vi "Convert_Data.vi"(0 "I2C_Data":T3 {"Target_Specification"."Target_Address" format="%x"; "Target_Specification"."Target_Type" items=["10 Bit Address", "7 Bit Address"]; "Target_Specification"."Register_Address" format="%x"; "Read_Write" items=["ADD TARGET"]}, 5 "CSV_String_In":string, 11 "Error_In":errorcluster, 13 "Convert_Mode":T5=enum."Data_to_String") -> (4 "I2C_Data":T3 {"Target_Specification"."Target_Address" format="%x"; "Target_Specification"."Target_Type" items=["10 Bit Address", "7 Bit Address"]; "Target_Specification"."Register_Address" format="%x"; "Read_Write" items=["ADD TARGET"]}, 6 "CSV_String":string, 8 "Data":T1[](array[typedef]) {"Target_Type" items=["10 Bit Address", "7 Bit Address"]; "Selected_Register_Address" format="%x"; "Target_Address" format="%x"}, 15 "Error_Out":errorcluster)   [LabVIEW 2023]
uses:
  Controls/Convert_Mode.ctl
  Class/I2C/I2C.lvclass
  Controls/Control 5.ctl
  Controls/Menu_Ring.ctl
  Controls/Control 2.ctl
  Controls/Converted_Data.ctl
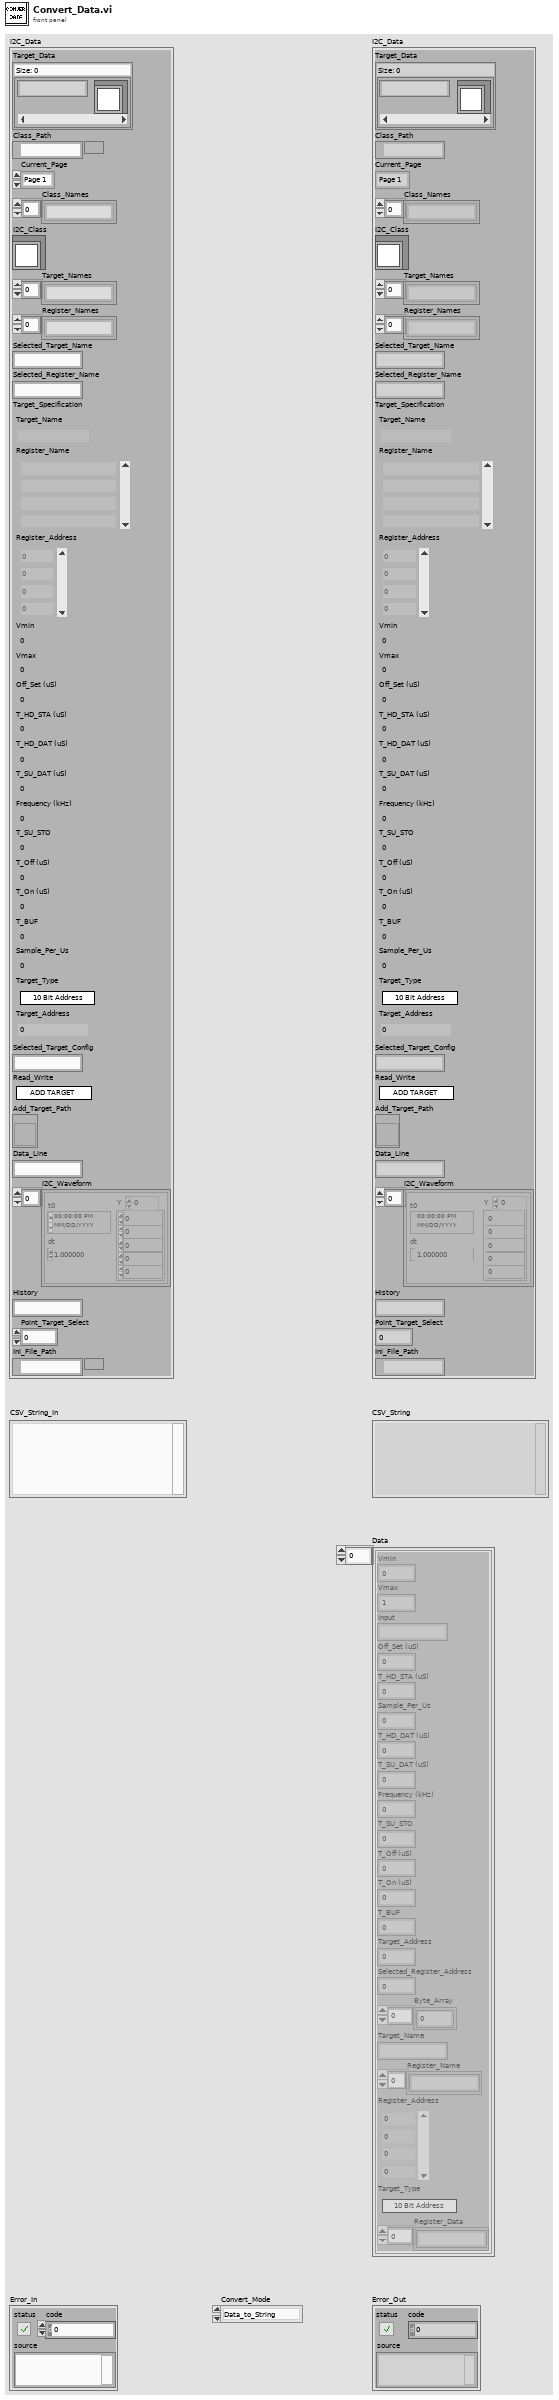
[diagram p1: front panel]
types:
  T1 = typedef "Converted_Data.ctl" = cluster{"Vmin":dbl, "Vmax":dbl, "Input":string, "Off_Set (uS)":dbl, "T_HD_STA (uS)":dbl, "Sample_Per_Us":dbl, "T_HD_DAT (uS)":dbl, "T_SU_DAT (uS)":dbl, "Frequency (kHz)":dbl, "T_SU_STO":dbl, "T_Off (uS)":dbl, "T_On (uS)":dbl, "T_BUF":dbl, "Target_Address":u16, "Selected_Register_Address":u8, "Byte_Array":u8[], "Target_Name":string, "Register_Name":string[], "Register_Address":u8[], "Target_Type":T2, "Register_Data":string[]}
  T2 = typedef "Menu_Ring.ctl" = u16
  T3 = typedef "Convert_Mode.ctl" = cluster{"Target_Data":map{string, refnum<class "I2C.lvclass">}, "Class_Path":path, "Current_Page":enum32{"Page 1", "Page 2"}, "Class_Names":string[], "I2C_Class":refnum<class "I2C.lvclass">, "Target_Names":string[], "Register_Names":string[], "Selected_Target_Name":string, "Selected_Register_Name":string, "Target_Specification":T4, "Selected_Target_Config":string, "Read_Write":T2, "Add_Target_Path":refnum<vi>, "Data_Line":string, "I2C_Waveform":waveform(dbl)[], "History":string, "Point_Target_Select":i32, "Ini_File_Path":path}
  T4 = typedef "Control 5.ctl" = cluster{"Target_Name":string, "Register_Name":string[], "Register_Address":u16[], "Vmin":dbl, "Vmax":dbl, "Off_Set (uS)":dbl, "T_HD_STA (uS)":dbl, "T_HD_DAT (uS)":dbl, "T_SU_DAT (uS)":dbl, "Frequency (kHz)":dbl, "T_SU_STO":dbl, "T_Off (uS)":dbl, "T_On (uS)":dbl, "T_BUF":dbl, "Sample_Per_Us":dbl, "Target_Type":T2, "Target_Address":u16}
  T5 = typedef "Control 2.ctl" = enum16{"String_To_Data", "Data_to_String"}
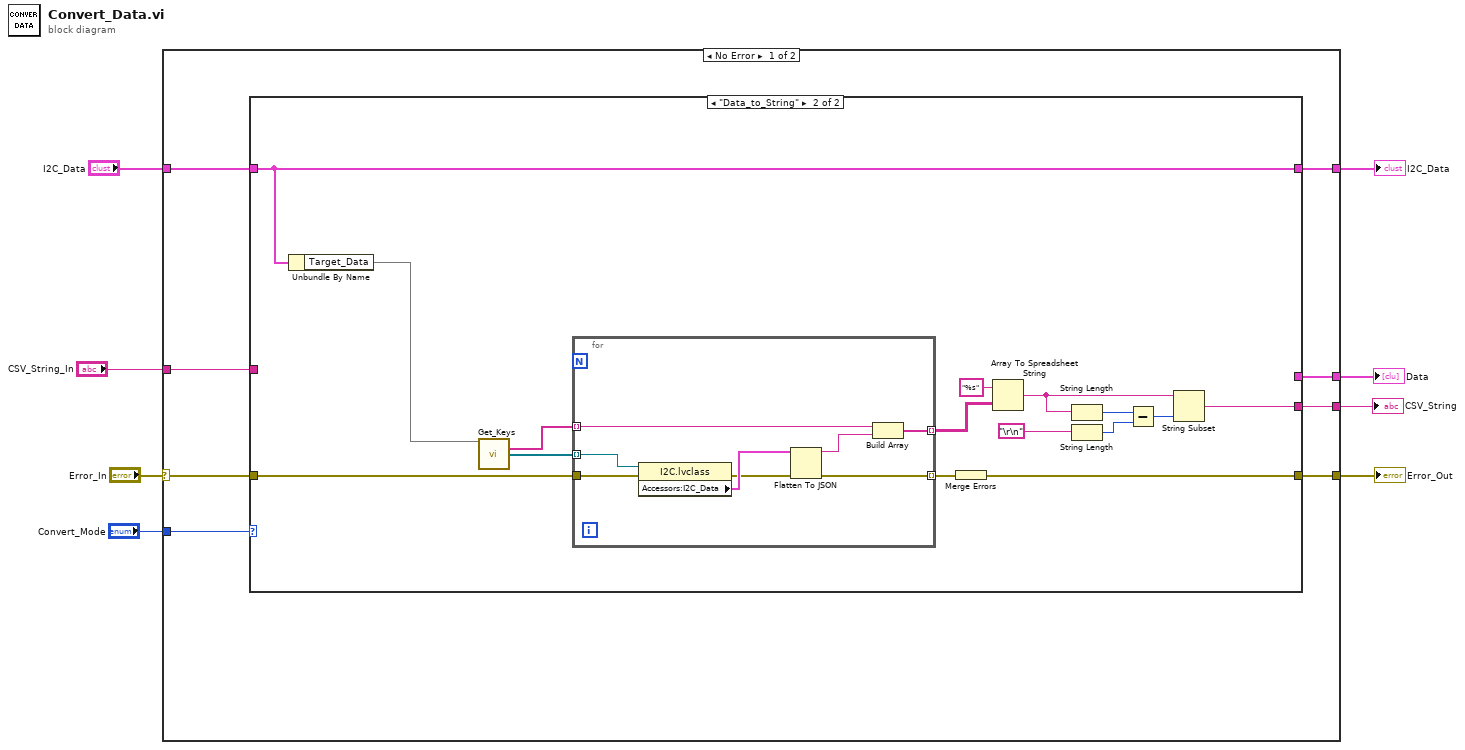
[diagram p0: block diagram]
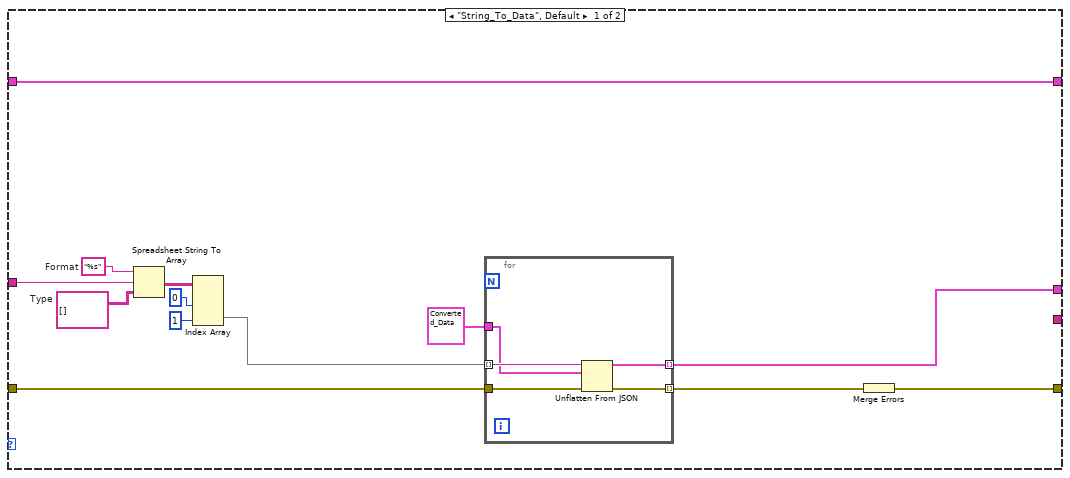
[diagram p2: hidden frame]
diagram:
  n1 = case shown="No Error" "Error_In" {
    selector: "Error_In" -> [w15 w59]
    tunnel: "I2C_Data" -> [w16 w58]
    tunnel: [w14 w59] -> w6
    tunnel: [w13 _] -> w5
    tunnel: "Convert_Mode" -> [w12 _]
    tunnel: "CSV_String_In" -> [w11 _]
    tunnel: [w10 w58] -> w2
    tunnel: [w9 _] -> w1
    frame No Error {
      n2 = case shown="\"Data_to_String\"" w12 {
        tunnel: w16 -> [w20 w37]
        tunnel: w15 -> [w18 w48]
        tunnel: [w25 w36] -> w14
        tunnel: [_ w38] -> w13
        tunnel: w11 -> [w29 _]
        tunnel: [w20 w37] -> w10
        tunnel: [w19 _] -> w9
        frame "String_To_Data", Default {
          w21 = string[][] []  # Type
          w28 = "%s"  # Format
          n3 = Spreadsheet String To Array(format string=w28, spreadsheet string=w29, array type (2D Dbl)=w21) -> (array=w27:string[][])  [unwired: 1 in]
          n4 = Index Array(array=w27, index (col) #1=0 ("disabled index (col)"), index (col) #2=1 ("index (col)")) -> (element #2=w24:string[])  [unwired: 2 in, 1 out]
          n5 = for {
            tunnel: w18 -> [w34]
            tunnel: [w32] -> w26 mode=indexing
            tunnel: w24 -> [w33] mode=indexing
            tunnel: [w31] -> w19 mode=indexing
            tunnel: T1 {"Vmin"=0.0, "Vmax"=1.0, "Input"="", "Off_Set (uS)"=0.0, "T_HD_STA (uS)"=0.0, "Sample_Per_Us"=0.0, "T_HD_DAT (uS)"=0.0, "T_SU_DAT (uS)"=0.0, "Frequency (kHz)"=0.0, "T_SU_STO"=0.0, "T_Off (uS)"=0.0, "T_On (uS)"=0.0, "T_BUF"=0.0, "Target_Address"=0, "Selected_Register_Address"=0, "Byte_Array"=[], "Target_Name"="", "Register_Name"=[], "Register_Address"=[], "Target_Type"=0, "Register_Data"=[]} ("I2C_Data") -> [w30]
            n6 = Unflatten From JSON(JSON string=w33, type and defaults=w30, error in (no error)=w34) -> (value=w31:T1, error out=w32:errorcluster)  [unwired: 4 in]
          }
          n7 = Merge Errors(w26) -> (w25:errorcluster)
        }
        frame "Data_to_String" {
          n8 = Unbundle By Name(w37) -> ("Target_Data"=w49:map{string, refnum<class "I2C.lvclass">})
          n9 = call "Get_Keys.vi"("Target_Data"=w49) -> ("Keys"=w40:string[], "Elements"=w35:refnum<class "I2C.lvclass">[])  [unwired: 10 in, 3 out]
          n10 = for {
            tunnel: w48 -> [w57]
            tunnel: [w51] -> w47 mode=indexing
            tunnel: w40 -> [w56] mode=indexing
            tunnel: [w55] -> w39 mode=indexing
            tunnel: w35 -> [w50] mode=indexing
            n11 = property class="I2C.lvclass"(reference=w50, error in=w57) -> (error out=w52:errorcluster, "Accessors:I2C_Data"=w54:T1)  [unwired: 1 out]
            n12 = Flatten To JSON(anything=w54, error in (no error)=w52) -> (JSON string=w53:string, 11:w51:errorcluster)  [unwired: 1 in]
            n13 = Build Array(w56, w53) -> (w55:string[])
          }
          n14 = Merge Errors(w47) -> (w36:errorcluster)
          n15 = Array To Spreadsheet String(array=w39, 3:"%s" ("format string")) -> (spreadsheet string=w42:string)  [unwired: 1 in]
          n16 = String Length(string=w42) -> (length=w44:i32)
          n17 = String Length(string="\r\n") -> (length=w43:i32)
          n18 = Subtract(x=w44, y=w43) -> (x-y=w41:i32)
          n19 = String Subset(string=w42, length (rest)=w41) -> (substring=w38:string)  [unwired: 1 in]
        }
      }
    }
    frame Error {
    }
  }
  "Error_Out" <- w6
  "CSV_String" <- w5
  "I2C_Data" <- w2
  "Data" <- w1
